vi "ToSGLfrom32bI4.vi"(8 "Input Valid":bool, 11 "FXP Input":fxp<+/-,32,3>) -> (0 "Output Valid":bool, 3 "Float Output":fxp<+,32,32>)   [LabVIEW 2012]
doc: "<b> Latency = 6 Ticks </b>"
uses:
  <vilib>/rvi/IPIntegrationNode/IPINode_Utilities/niFpgaIPINodeSimCore.vi
  <vilib>/rvi/FXPMathLib/basic elements/FxpDiscreteDelay/XNode/nifxpmath_DiscreteDelay.xnode
  <vilib>/rvi/XilinxIP/XIPIN_XNode/niFpgaXIPIN.xnode
  <userlib>/FPGA Library/Code Development/SGL/Conversions/ToSGLfrom32b/ToSGLfrom32bI4/ToSGLfrom32bI3/ToSGLfrom32bI3_89D7124B462088804037CDBBE1B1C172.dll
  <vilib>/rvi/IPIntegrationNode/IPINode_Xnode/niFpgaIPINode.xnode
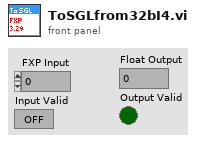
[diagram p1: front panel]
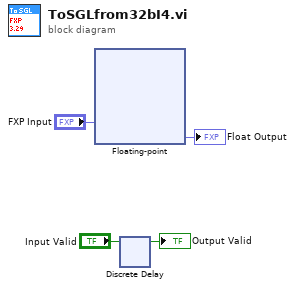
[diagram p0: block diagram]
diagram:
  n1 = xnode ("Floating-point")("a"="FXP Input") -> ("result"=→"Float Output":fxp<+,32,32>)
  n2 = xnode "Discrete Delay"("D"="Input Valid") -> ("Q"=→"Output Valid":bool)
